vi "globals.vi"() -> ()   [LabVIEW 2015]
panel:
  out "Lifted":bool
  out "Lowered":bool
  out "Shoulder angle":dbl
  out "Elbow angle":dbl
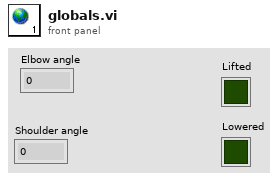
[diagram p1: front panel]
diagram:
